vi "Assignment3_2.vi"() -> ()   [LabVIEW 2025]
doc: "This VI is a StopWatch where you can start, pause, resume, reset and stop"
uses:
  TypeDef/States.ctl
panel:
  in  "PAUSE":bool
  out "MilliSeconds(ms)":dbl
  out "Seconds(s)":dbl
  out "Minute(min)":dbl
  out "Hour(hr)":dbl
  in  "STOP":bool
  in  "RESUME":bool
  in  "RESET":bool
  in  "START":bool
  # "STOPWATCH"
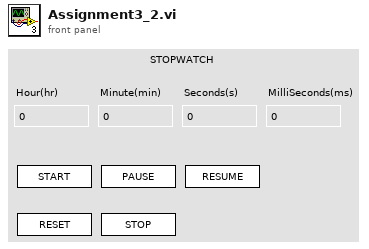
[diagram p1: front panel]
types:
  T1 = typedef "States.ctl" = enum16{"DoNothing", "START", "PAUSED"}
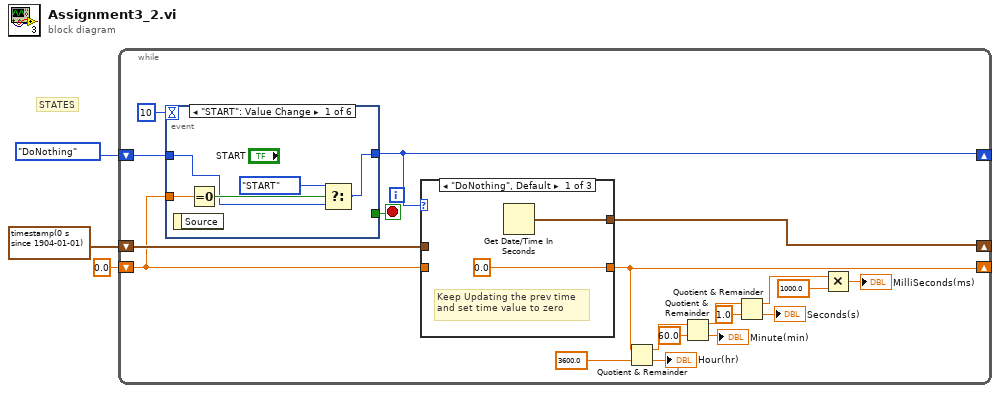
[diagram p0: block diagram]
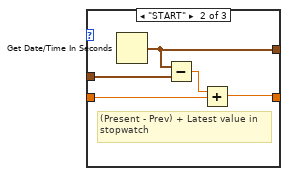
[diagram p2: hidden frame]
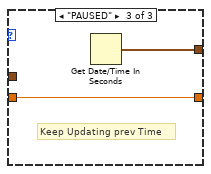
[diagram p3: hidden frame]
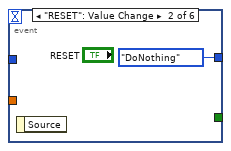
[diagram p4: hidden frame]
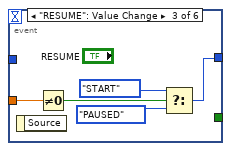
[diagram p5: hidden frame]
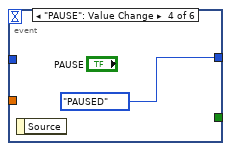
[diagram p6: hidden frame]
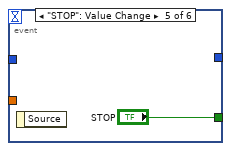
[diagram p7: hidden frame]
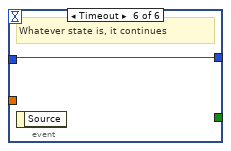
[diagram p8: hidden frame]
diagram:
  # "STATES"
  n1 = while {
    shift-right: [w18] -> _
    shift-left: timestamp(0 s since 1904-01-01) ("seconds since 1Jan1904") -> [w17]
    shift-right: [w20] -> _
    shift-left: States."DoNothing" -> [w19]
    shift-right: [w16] -> _
    shift-left: 0.0 -> [w4]
    stop <- w22 stop-if-true
    n2 = event shown="[0] \"START\": Value Change" {
      selector: _ -> [_ _ _ _ _ _]
      dyn-events: _ -> [_ _ _ _ _ _]
      timeout: 10 -> [_ _ _ _ _ _]
      tunnel: [_ _ _ _ "STOP" _] -> w22
      tunnel: [w33 States."DoNothing" w38 States."PAUSED" ("Enum") _ w45] -> w20
      tunnel: w19 -> [w32 _ _ _ _ w45]
      tunnel: w4 -> [w36 _ w42 _ _ _]
      event "START": Value Change {
        n3 = event-data() -> ()  [unwired: 1 in, 1 out]
        n4 = Equal To 0?(x=w36) -> (x = 0?=w35:bool)
        n5 = Select(t=States."START", s=w35, f=w32) -> (s? t:f=w33:T1)
      }
      event "RESET": Value Change {
        n6 = event-data() -> ()  [unwired: 1 in, 1 out]
      }
      event "RESUME": Value Change {
        n7 = event-data() -> ()  [unwired: 1 in, 1 out]
        n8 = Not Equal To 0?(x=w42) -> (x != 0?=w41:bool)
        n9 = Select(t=States."START", s=w41, f=States."PAUSED" ("Enum")) -> (s? t:f=w38:T1)
      }
      event "PAUSE": Value Change {
        n10 = event-data() -> ()  [unwired: 1 in, 1 out]
      }
      event "STOP": Value Change {
        n11 = event-data() -> ()  [unwired: 1 in, 1 out]
      }
      event Timeout {
        # "Whatever state is, it continues"
        n12 = event-data() -> ()  [unwired: 1 in, 1 out]
      }
    }
    n13 = case shown="\"DoNothing\", Default" w20 {
      tunnel: w4 -> [_ w27 w31]
      tunnel: [0.0 ("t") w25 w31] -> w16
      tunnel: [w23 w26 w30] -> w18
      tunnel: w17 -> [_ w29 _]
      frame "DoNothing", Default {
        # "Keep Updating the prev time\nand set time value to zero"
        n14 = Get Date/Time In Seconds() -> (seconds since 1Jan1904=w23:timestamp)
      }
      frame "START" {
        # "(Present - Prev) + Latest value in\nstopwatch"
        n15 = Get Date/Time In Seconds() -> (seconds since 1Jan1904=w26:timestamp)
        n16 = Subtract(x=w26, y=w29) -> (x-y=w28:dbl)
        n17 = Add(x=w28, y=w27) -> (x+y=w25:dbl)
      }
      frame "PAUSED" {
        # "Keep Updating prev Time"
        n18 = Get Date/Time In Seconds() -> (seconds since 1Jan1904=w30:timestamp)
      }
    }
    n19 = Quotient & Remainder(x=w16, y=3600.0) -> (x-y*floor(x/y)=w13:dbl, floor(x/y)=→"Hour(hr)":dbl)
    n20 = Quotient & Remainder(x=w13, y=60.0) -> (x-y*floor(x/y)=w6:dbl, floor(x/y)=→"Minute(min)":dbl)
    n21 = Quotient & Remainder(x=w6, y=1.0) -> (x-y*floor(x/y)=w7:dbl, floor(x/y)=→"Seconds(s)":dbl)
    n22 = Multiply(x=w7, y=1000.0) -> (x*y=→"MilliSeconds(ms)":dbl)
  }
